vi "Init.vi"(8 "error in (no error)":errorcluster, 11 "Data Sharing Plugin Runtime in":refnum<class "Plugin Runtime.lvclass">) -> (0 "error out":errorcluster, 3 "Data Sharing Plugin Runtime out":refnum<class "Plugin Runtime.lvclass">)   [LabVIEW 2016, in "Plugin Runtime.lvclass"]
uses:
  Plugin Runtime.lvclass
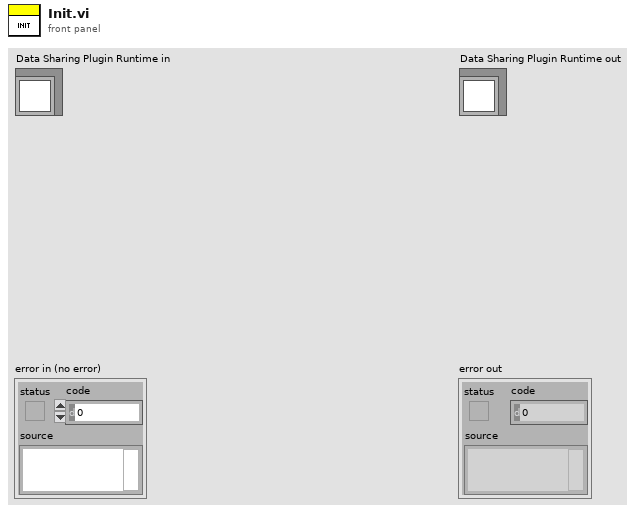
[diagram p1: front panel]
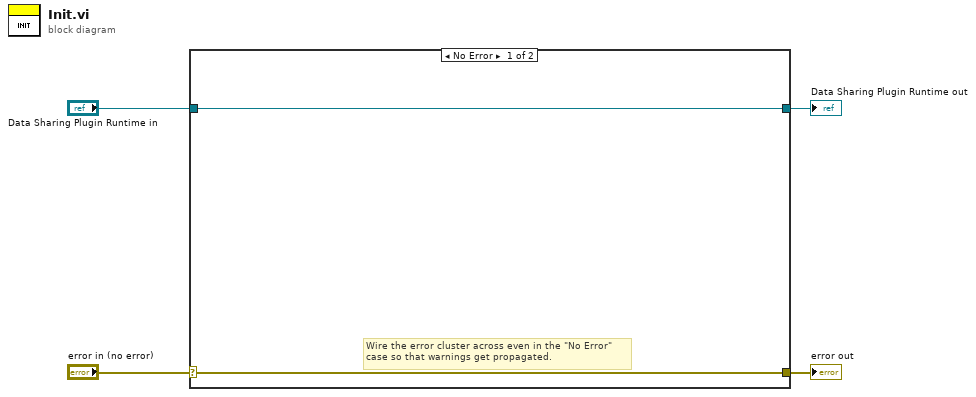
[diagram p0: block diagram]
diagram:
  n1 = case shown="No Error" "error in (no error)" {
    selector: "error in (no error)" -> [w5 w8]
    tunnel: [w5 w8] -> w3
    tunnel: [w6 w7] -> w1
    tunnel: "Data Sharing Plugin Runtime in" -> [w6 w7]
    frame No Error {
      # "Wire the error cluster across even in the \"No Error\"\ncase so that warnings get propagated."
    }
    frame Error {
    }
  }
  "error out" <- w3
  "Data Sharing Plugin Runtime out" <- w1
